vi "Zones layout drawing test with smoothing and edge detection.vi"() -> ()   [LabVIEW 2018]
uses:
  Tracker.lvlib
  SubVi's/Controls/CTL_Draw_Area_Size.ctl
panel:
  in  "Preserve size? (F)":bool
  in  "Edge output? (F)":bool
  in  "Edge detection weight parameter":dbl(slide)=16.0 min=0.01 max=128.0 scale=0.001..100.0
  out "x-y":dbl
  out "size(s) 2":i32[](array[numeric])
  out "size(s)":i32[](array[numeric])
  out "Experiment Diagram 2":T1(plugin-control)
  in  "Draw Area Size (480x480)":T2={"Width"=480, "Height"=480}
  out "Experiment Diagram 1a":T1(plugin-control)
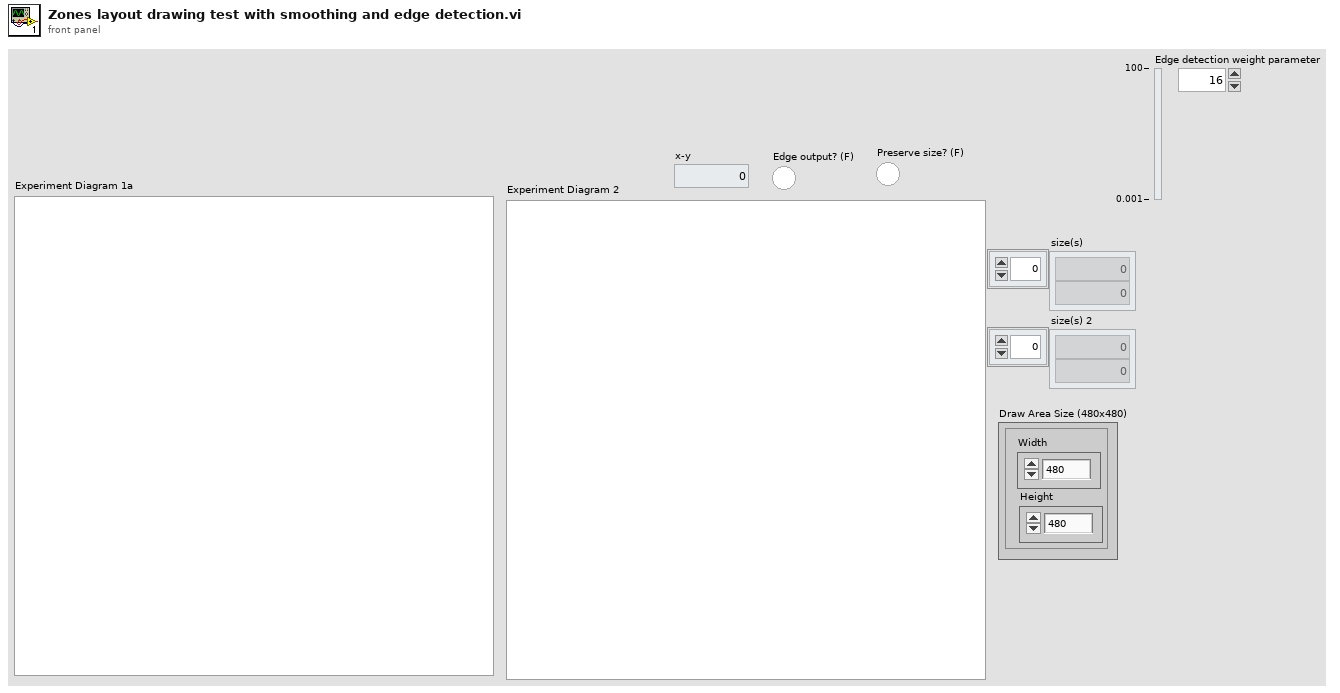
[diagram p1: front panel]
types:
  T1 = typedef "IMAQ Image.ctl" = refnum<image>
  T2 = typedef "Tracker.lvlib/CTL_Draw_Area_Size.ctl" = cluster{"Width":i32, "Height":i32}
  T3 = typedef "Image Type" = u32
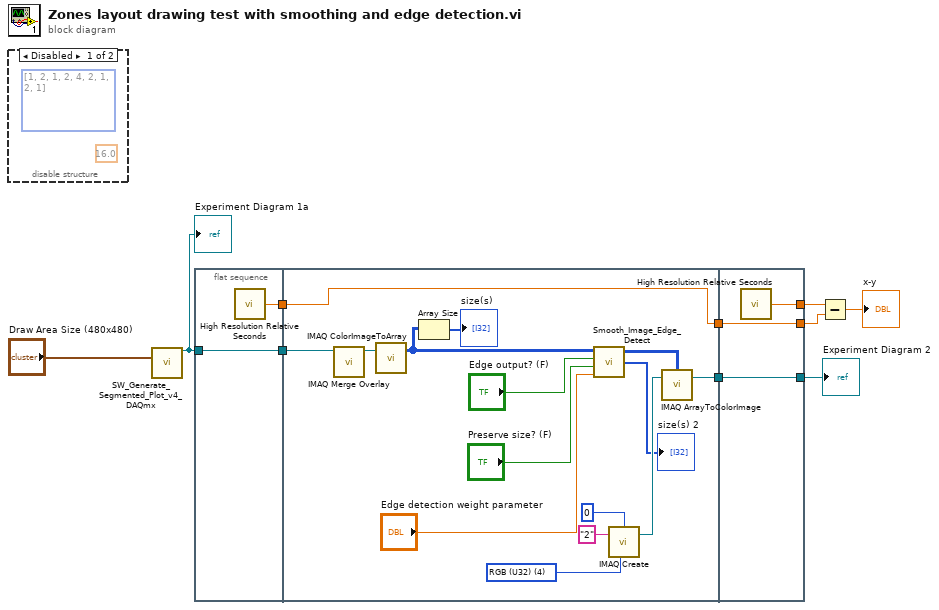
[diagram p0: block diagram]
diagram:
  n1 = disable-structure shown="Disabled" {
    frame Disabled {
      (unwired) 16.0
      w11 = i32[][] [[1, 2, 1], [2, 4, 2], [1, 2, 1]]
    }
    frame Enabled {
    }
  }
  n2 = call "SW_Generate_Segmented_Plot_v4_DAQmx.vi"("Draw Area Size (480x480)"="Draw Area Size (480x480)") -> ("Experiment Diagram"=w9:T1)  [unwired: 8 in, 6 out]
  "Experiment Diagram 1a" <- w9
  n3 = flat-sequence {
    tunnel: w9 -> [w13]
    tunnel: [w13] -> w7
    tunnel: [w12] -> w3
    tunnel: w7 -> [w21]
    tunnel: [w27] -> w6
    tunnel: w3 -> [w18]
    tunnel: [w18] -> w1
    tunnel: [w31] -> w10
    tunnel: w6 -> [w31]
    tunnel: [w30] -> w5
    tunnel: [w29] -> w2
    tunnel: w1 -> [w29]
    frame #0 {
      n4 = call <vilib>:"High Resolution Relative Seconds.vi"() -> ("relative seconds"=w12:dbl)
    }
    frame #1 {
      w24 = T3 4 items=["Grayscale (U8)", "Grayscale (I16)", "Grayscale (SGL)", "Complex (CSG)", "RGB (U32)", "HSL (U32)", "RGB (U64)", "Grayscale (U16)"] ("Image Type")
      n5 = call "IMAQ Merge Overlay"("Image Src"=w21) -> ("Image Dst Out"=w28:T1)  [unwired: 9 in, 1 out]
      n6 = call "IMAQ ColorImageToArray"("Image"=w28) -> ("Image Pixels (U32)"=w20:u32[][])  [unwired: 3 in, 2 out]
      n7 = Array Size(array=w20) -> (size(s)=→"size(s)":i32[])
      n8 = call "Smooth_Image_Edge_Detect.vi"("Edge detection weight parameter"="Edge detection weight parameter", "Preserve size? (F)"="Preserve size? (F)", "Edge output? (F)"="Edge output? (F)", "Input Image Pixels (U32)"=w20) -> ("Output image size"=→"size(s) 2":i32[], "Output Image Pixels (U32)"=w19:u32[][])  [unwired: 1 in]
      n9 = call "IMAQ Create"("Border Size"=0, "Image Name"="2", "Image Type"=w24) -> ("New Image"=w26:T1)  [unwired: 2 in, 1 out]
      n10 = call "IMAQ ArrayToColorImage"("Image Pixels (U32)"=w19, "Image"=w26) -> ("Image Out"=w27:T1)  [unwired: 3 in, 1 out]
    }
    frame #2 {
      n11 = call <vilib>:"High Resolution Relative Seconds.vi"() -> ("relative seconds"=w30:dbl)
    }
  }
  n12 = Subtract(x=w5, y=w2) -> (x-y=→"x-y":dbl)
  "Experiment Diagram 2" <- w10
